vi "Import MTL.vi"(8 "error in (no error)":errorcluster, 11 "Material":path) -> (0 "error out":errorcluster, 3 "Material":T1)   [LabVIEW 2020, in "3D.lvlib"]
uses:
  3D.lvlib
  Material.ctl
  Raster/Texture.ctl
  Raster/Rectangle Dimensions.ctl
  Raster/Raster.lvlib
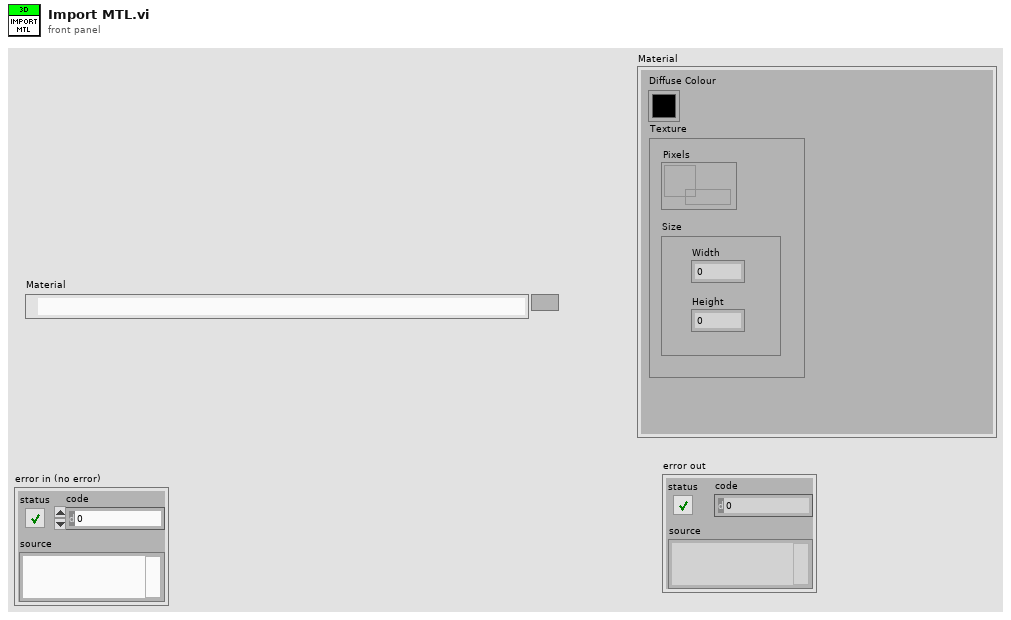
[diagram p1: front panel]
types:
  T1 = typedef "3D.lvlib/Material.ctl" = cluster{"Diffuse Colour":u32, "Texture":T2}
  T2 = typedef "Raster.lvlib/Texture.ctl" = cluster{"Pixels":refnum<data-value>, "Size":T3}
  T3 = typedef "Raster.lvlib/Rectangle Dimensions.ctl" = cluster{"Width":u32, "Height":u32}
  T4 = typedef "imagedata.ctl" = cluster{"image type":i32, "image depth":i32, "image":u8[], "mask":u8[], "colors":u32[], "Rectangle":cluster{"left":i16, "top":i16, "right":i16, "bottom":i16}}
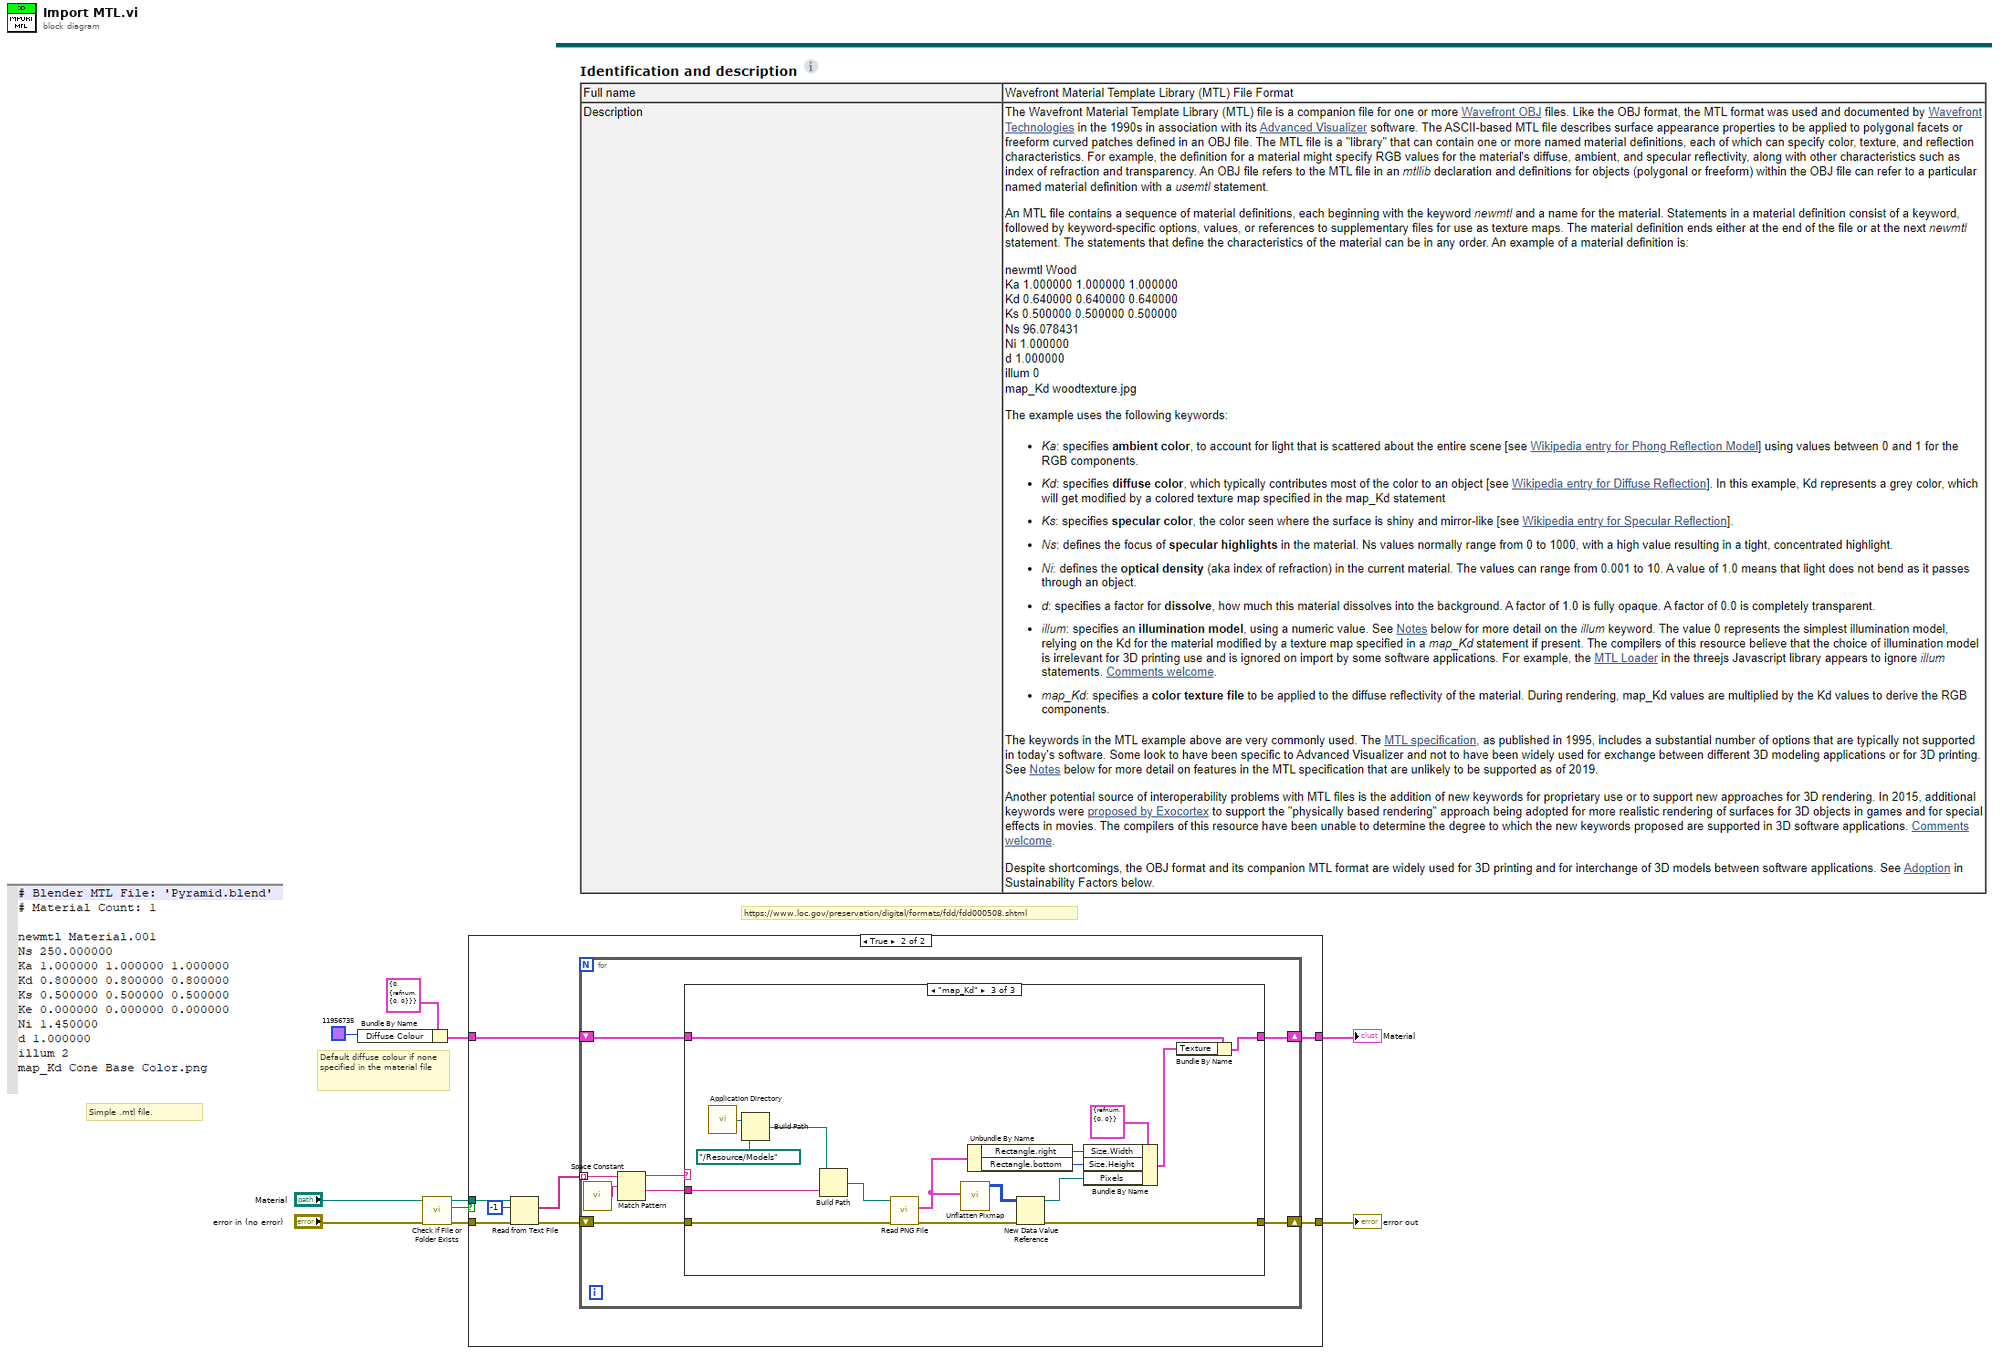
[diagram p0: block diagram]
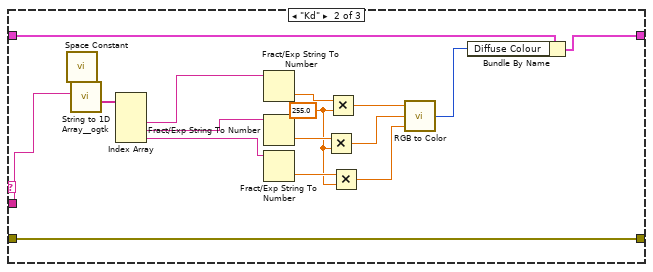
[diagram p4: hidden frame]
diagram:
  # "Default diffuse colour if none specified in the material file"
  # "https://www.loc.gov/preservation/digital/formats/fdd/fdd000508.shtml"
  # "Simple .mtl file."
  n1 = Bundle By Name(cluster=T1 {"Diffuse Colour"=0, "Texture"={"Pixels"=refnum, "Size"={"Width"=0, "Height"=0}}} ("Material"), "Diffuse Colour"=u32 11956735 ("s? t:f")) -> (w9:T1)
  n2 = call <vilib>:"Check if File or Folder Exists.vi"("error in (no error)"="error in (no error)", "path"="Material") -> ("error out"=w3:errorcluster, "file or folder exists?"=w1:bool, "dup path"=w2:path)  [unwired: 7 in]
  n3 = case shown="True" w1 {
    tunnel: w9 -> [w11 w17]
    tunnel: [w12 w16] -> w7
    tunnel: [w11 w15] -> w6
    tunnel: w3 -> [w12 w14]
    tunnel: w2 -> [_ w13]
    frame False {
    }
    frame True {
      n4 = Read from Text File(file (use dialog)=w13, count=-1, error in=w14) -> (text=w19:string[], error out=w18:errorcluster)  [unwired: 1 in, 2 out]
      n5 = for {
        tunnel: w19 -> [w24] mode=indexing
        shift-right: [w25] -> w16
        shift-left: w18 -> [w26]
        shift-right: [w27] -> w15
        shift-left: w17 -> [w28]
        n6 = call <vilib>:"Space Constant.vi"() -> ("String"=w23:string)
        n7 = Match Pattern(string=w24, regular expression=w23) -> (before substring=w22:string, after substring=w21:string)  [unwired: 1 in, 2 out]
        n8 = case shown="\"map_Kd\"" w22 {
          tunnel: w28 -> [w30 w40 w64]
          tunnel: [w30 w38 w63] -> w27
          tunnel: w26 -> [w29 w37 w53]
          tunnel: [w29 w37 w51] -> w25
          tunnel: w21 -> [_ w31 w48]
          frame Default {
          }
          frame "Kd" {
            w41 = 255.0 ("y")
            n9 = call <vilib>:"Space Constant.vi"() -> ("String"=w36:string)
            n10 = call <userlib>:"String to 1D Array__ogtk.vi"("delimiter (Tab)"=w36, "string"=w31) -> ("Array of Strings"=w35:string[])  [unwired: 9 in]
            n11 = Index Array(array=w35) -> (element #2=w34:string, element #3=w33:string, element #4=w32:string)  [unwired: 4 in, 1 out]
            n12 = Fract/Exp String To Number(string=w34) -> (number=w42:dbl)  [unwired: 3 in, 1 out]
            n13 = Fract/Exp String To Number(string=w33) -> (number=w43:dbl)  [unwired: 3 in, 1 out]
            n14 = Fract/Exp String To Number(string=w32) -> (number=w44:dbl)  [unwired: 3 in, 1 out]
            n15 = Multiply(x=w43, y=w41) -> (x*y=w46:dbl)
            n16 = Multiply(x=w42, y=w41) -> (x*y=w45:dbl)
            n17 = Multiply(x=w44, y=w41) -> (x*y=w47:dbl)
            n18 = call <vilib>:"RGB to Color.vi"("B"=w47, "G"=w46, "R"=w45) -> ("Color"=w39:u32)
            n19 = Bundle By Name(cluster=w40, "Diffuse Colour"=w39) -> (w38:T1)
          }
          frame "map_Kd" {
            n20 = call <vilib>:"Application Directory.vi"() -> ("Application Directory"=w61:path)
            n21 = Build Path(base path=w61, name or relative path=path "../Resource/Models") -> (appended path=w62:path)
            n22 = Build Path(base path=w62, name or relative path=w48) -> (appended path=w49:path)
            n23 = call <vilib>:"Read PNG File.vi"("error in (no error)"=w53, "path to PNG file"=w49) -> ("error out"=w52:errorcluster, "image data"=w56:T4)  [unwired: 7 in, 1 out]
            n24 = call <vilib>:"Unflatten Pixmap.vi"("image data"=w56) -> ("24-bit pixmap"=w55:u32[][])  [unwired: 4 in, 6 out]
            n25 = Unbundle By Name(w56) -> ("Rectangle.right"=w57:i16, "Rectangle.bottom"=w58:i16)
            n26 = New Data Value Reference(data value=w55, error in=w52) -> (data value reference=w59:refnum<data-value>, error out=w51:errorcluster)
            n27 = Bundle By Name(cluster=T2 {"Pixels"=refnum, "Size"={"Width"=0, "Height"=0}} ("Texture"), "Size.Width"=w57, "Size.Height"=w58, "Pixels"=w59) -> (w50:T2)
            n28 = Bundle By Name(cluster=w64, "Texture"=w50) -> (w63:T1)
          }
        }
      }
    }
  }
  "error out" <- w7
  "Material" <- w6
